vi "FitParabola (SubVI).vi"(0 "Normalized Intensity vs Radius in":cluster{dbl[], dbl[]}, 1 "x values":dbl[](array[numeric]), 2 "y values":dbl[](array[numeric]), 3 "Estimated mean":dbl, 4 "Estimated width":dbl, 7 "Nsigma Low":dbl=4.0 format="%#_13g", 8 "Use all points":bool, 9 "Nsigma High":dbl=4.0 format="%#_13g") -> (14 "data plot":cluster{dbl[], dbl[]}(graph), 15 "derivative data plot with Gaussian fit":T1(graph), 16 "Polynomial Coefficients":dbl[](array[numeric]), 17 "error":i32, 19 "residue":dbl)   [LabVIEW 2016]
uses:
  <vilib>/Analysis/6fits.llb/Curve Fitting Criteria.ctl
  <vilib>/Analysis/NI_AALPro.lvlib
panel:
  # "RESULTS"
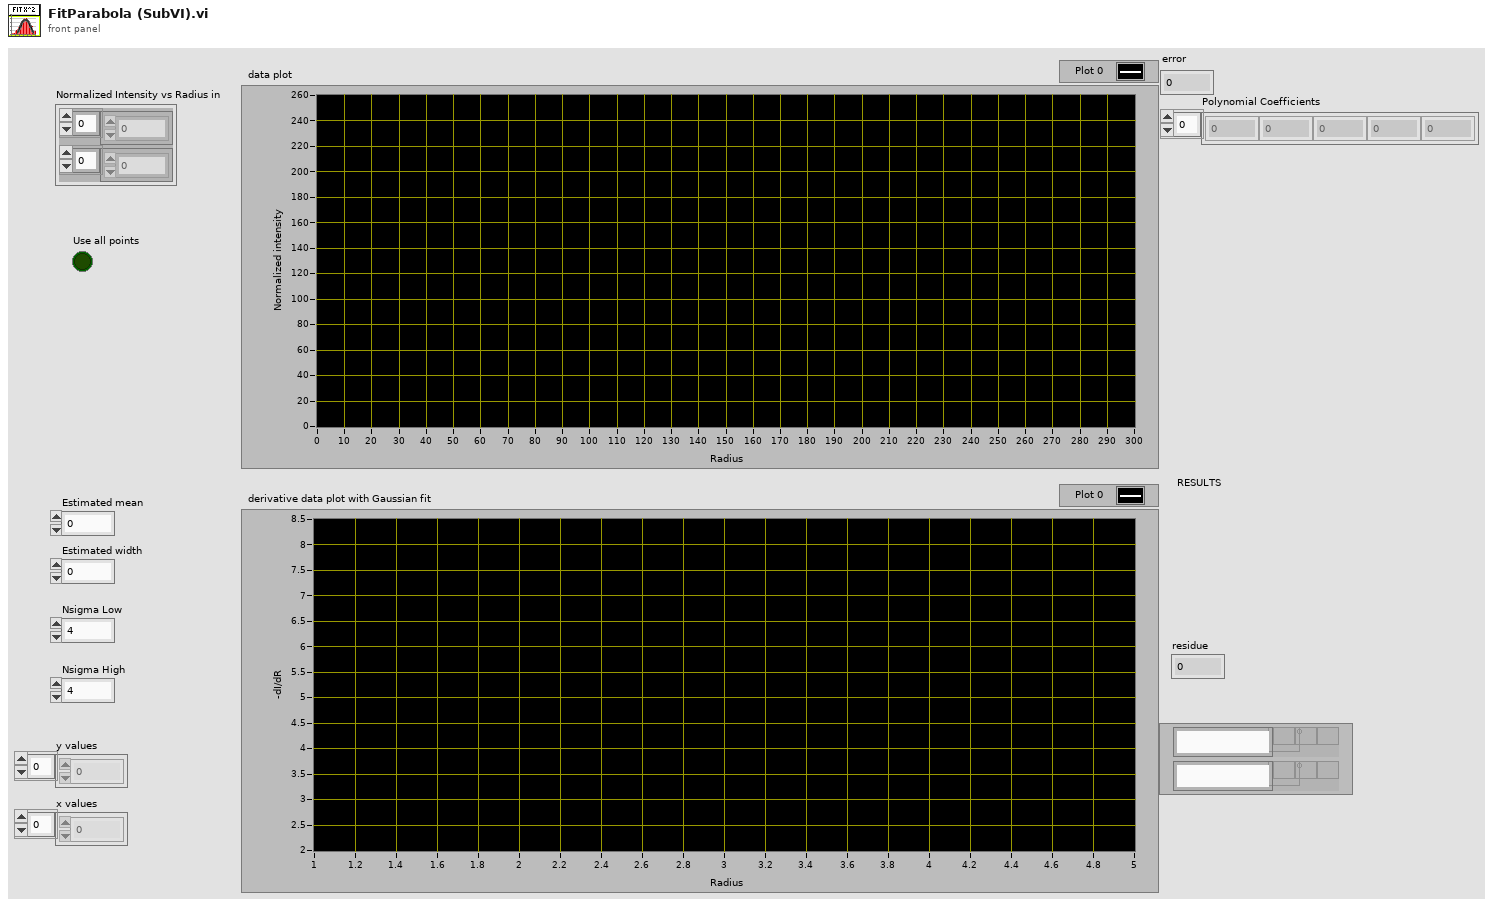
[diagram p1: front panel]
types:
  T1 = cluster{"Radius bins":dbl[], "Best Gaussian Fit":dbl[]}[]
  T2 = typedef "NI_AALPro.lvlib/Curve Fitting Criteria.ctl" = u16
  T3 = cluster{"x values":dbl[], "Best Polynomial Fit":dbl[]}
  T4 = cluster{"x values":dbl[], "Best Polynomial Fit":dbl[]}[]
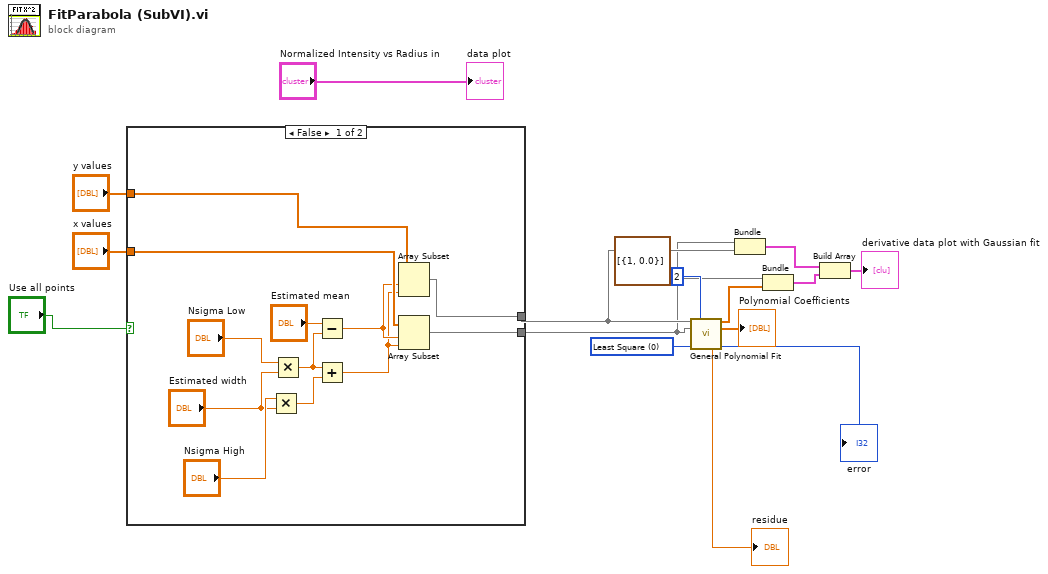
[diagram p0: block diagram]
diagram:
  w4 = T2 0 items=["Least Square", "Least Absolute Residual", "Bisquare"] ("method")
  (unwired) cluster{"order":i32, "coefficient":dbl}[] [{"order"=1, "coefficient"=0.0}] ("Coefficient Constraint")
  n1 = case shown="False" "Use all points" {
    tunnel: "y values" -> [w25 w28]
    tunnel: [w24 w28] -> w6
    tunnel: "x values" -> [w23 w29]
    tunnel: [w22 w29] -> w5
    frame False {
      n2 = Multiply(x="Nsigma High", y="Estimated width") -> (x*y=w17:dbl)
      n3 = Multiply(x="Nsigma Low", y="Estimated width") -> (x*y=w18:dbl)
      n4 = Subtract(x="Estimated mean", y=w18) -> (x-y=w21:dbl)
      n5 = Add(x=w18, y=w17) -> (x+y=w16:dbl)
      n6 = Array Subset(array=w25, index=w21, length=w16) -> (w24:dbl[])
      n7 = Array Subset(array=w23, index=w21, length=w16) -> (w22:dbl[])
    }
    frame True {
    }
  }
  n8 = call <vilib>:"General Polynomial Fit.vi"("Y"=w6, "polynomial order"=2, "X"=w5, "method"=w4) -> ("Best Polynomial Fit"=w14:dbl[], "Polynomial Coefficients"=→"Polynomial Coefficients":dbl[], "residue"=→"residue":dbl, "error"=→"error":i32)  [unwired: 8 in]
  n9 = Bundle("x values"=w5, "y values"=w6) -> (w9:cluster{"x values":dbl[], "y values":dbl[]})  [unwired: 1 in]
  n10 = Bundle("x values"=w5, "Best Polynomial Fit"=w14) -> (w13:T3)  [unwired: 1 in]
  n11 = Build Array(w9, w13) -> (→"derivative data plot with Gaussian fit":T4)
  "data plot" <- "Normalized Intensity vs Radius in"
